vi "Actor Core.vi"(8 "error in":errorcluster, 11 "Analog Output Channel in":refnum<class "Analog Output Channel.lvclass">) -> (0 "error out":errorcluster, 3 "Actor out":refnum<class "Actor.lvclass">)   [LabVIEW 2015, in "Analog Output Channel.lvlib" / "Analog Output Channel.lvclass"]
doc: "(<B>Filename</B>: Actor Framework.lvlib:Actor.lvclass:Actor Core.vi)\n\nReceives messages to the actor, reacts to them, and initiates any error handling that may shut the actor down.\n\nDescendant classes may override this VI to append parallel tasks for the actor to complete while it handles messages. Overrides use the Call Parent Method node."
uses:
  Analog Output Channel.lvclass
  <vilib>/ActorFramework/Actor/Actor.lvclass
  <vilib>/ActorFramework/Actor/Actor.lvclass/Actor.ctl
  <vilib>/ActorFramework/Message Enqueuer/Message Enqueuer.lvclass/Message Enqueuer.ctl
  <userlib>/_Win8uiFramework/ViewableActor.lvclass/ViewableActor.ctl
  AOChData.lvclass
  <userlib>/_Win8uiFramework/Read Stop Event.vi
  <vilib>/ActorFramework/Message Enqueuer/Init from Existing Queue.vi
  <vilib>/ActorFramework/Message Enqueuer/Message Enqueuer.lvclass
  Channel/ChannelInfo.lvclass
  Channel/ChannelData.lvclass
  Channel/ChannelConfig.lvclass
  Output Channel/Output Channel/Output Channel.lvclass
  <userlib>/_Win8uiFramework/ViewableActor.lvclass
  <userlib>/_Win8uiFramework/Win8uiFramework.lvlib
  Analog Output Channel Messages/Write Sine Wave Msg/Write Sine Wave Msg.lvclass
panel:
  out "size(s)":i32
  in  "String":string
  out "Waveform Graph":dbl[](graph)
  in  "Write Sine Wave":bool
  in  "Sine Wave Parameters":T1={"phase"=0.0, "amplitude"=1.0, "frequency"=10.0, "offset"=0.0} {"offset" format="%#_13g"; "frequency" format="%0.2p"; "amplitude" format="%0.2p"; "phase" format="%.2p"}
  out "Sequence Parameters":cluster{"Buffer Size":dbl, "Sample Rate":dbl}
  out "Device Address":tag
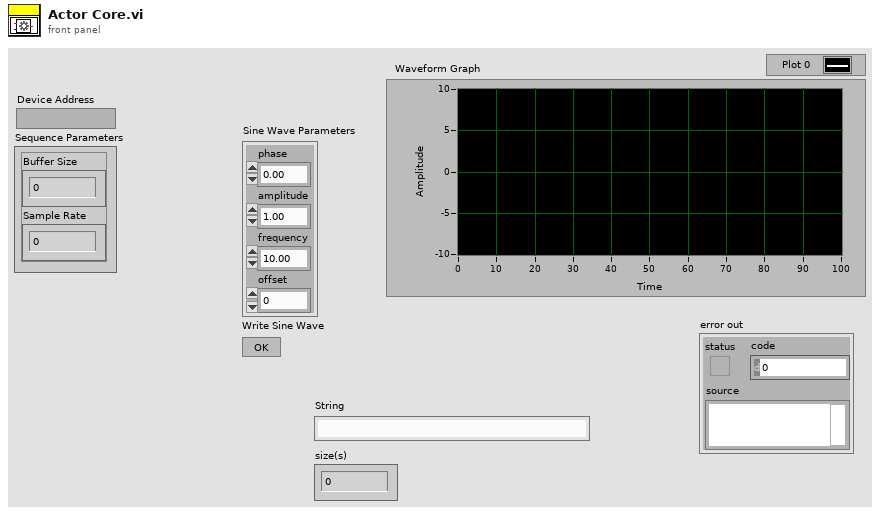
[diagram p1: front panel]
types:
  T1 = cluster{"phase":dbl, "amplitude":dbl, "frequency":dbl, "offset":dbl}
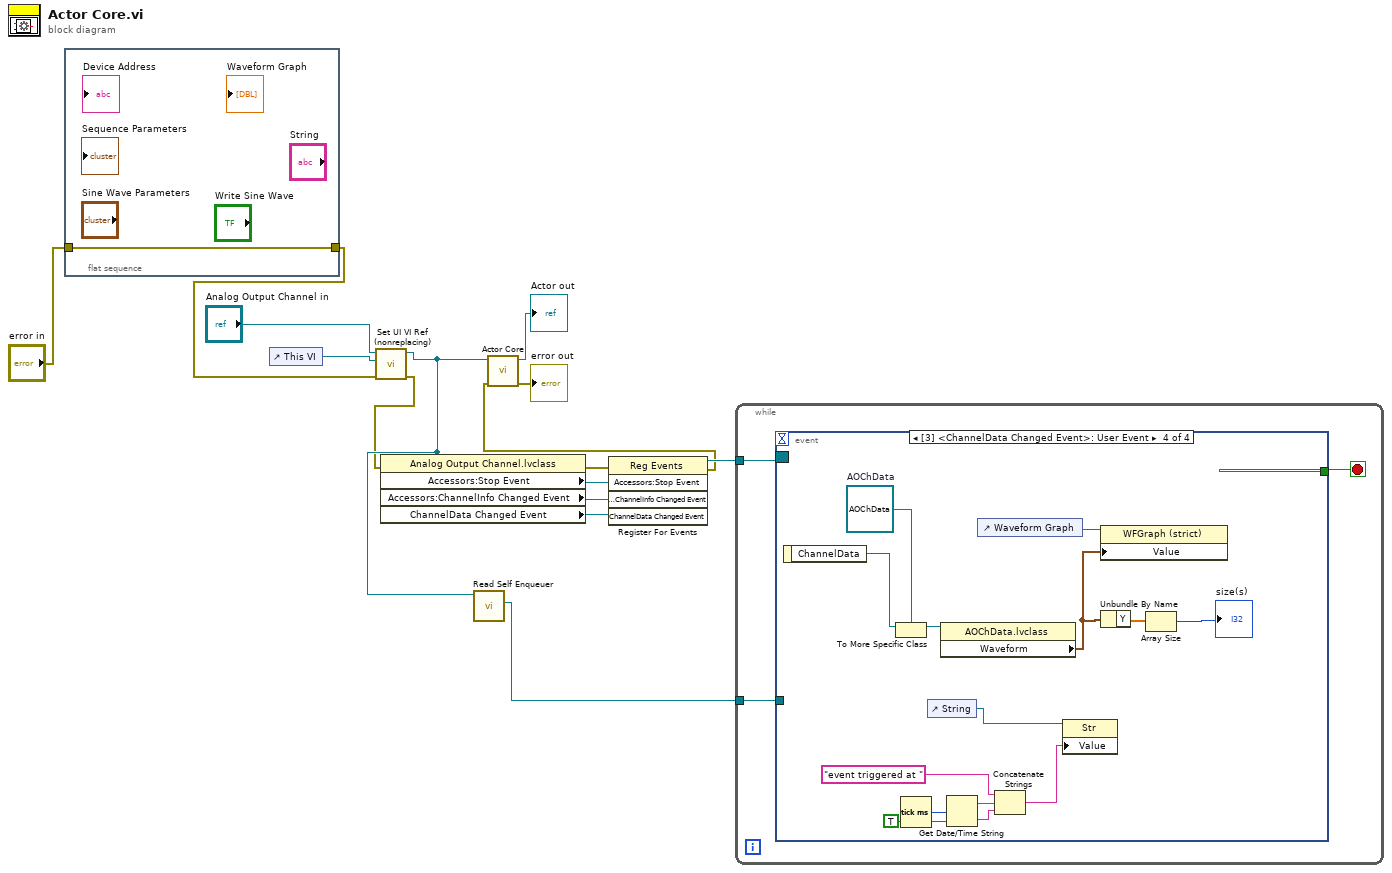
[diagram p0: block diagram]
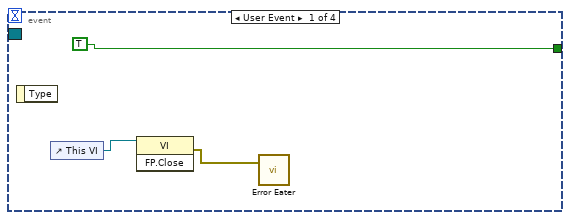
[diagram p2: hidden frame]
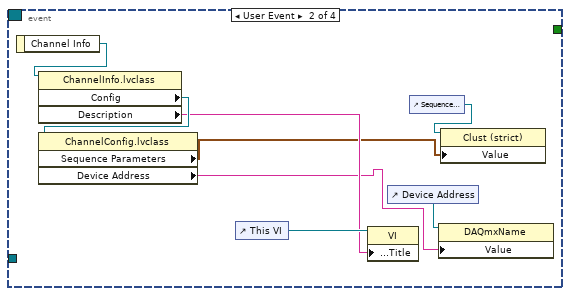
[diagram p3: hidden frame]
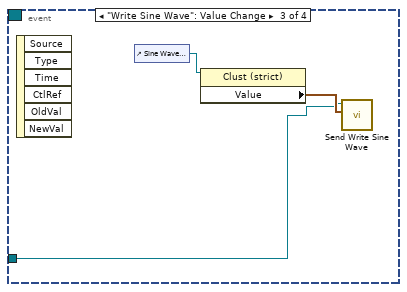
[diagram p4: hidden frame]
diagram:
  n1 = flat-sequence {
    tunnel: "error in" -> [w16]
    tunnel: [w16] -> w1
    frame #0 {
    }
  }
  n2 = control-ref of="This VI"() -> (w13:refnum<vi>)
  n3 = call <userlib>:"Set UI VI Ref (nonreplacing).vi"("error in (no error)"=w1, "UI VI Ref"=w13, "ViewableActor in"="Analog Output Channel in") -> ("error out"=w5:errorcluster, "ViewableActor out"=w8:refnum<class "Analog Output Channel.lvclass">)  [unwired: 6 in, 1 out]
  n4 = property class="Analog Output Channel.lvclass"(reference=w8, error in=w5) -> (error out=w4:errorcluster, "Accessors:Stop Event"=w11:refnum<user-event>, "Accessors:ChannelInfo Changed Event"=w10:refnum<user-event>, "ChannelData Changed Event"=w6:refnum<user-event>)  [unwired: 1 out]
  n5 = call <vilib>:"Read Self Enqueuer.vi"("Actor"=w8) -> ("Self Enqueuer"=w7:refnum<class "Message Enqueuer.lvclass">)  [unwired: 10 in]
  n6 = register-events(error in=w4, w11, w10, w6) -> (reference out=w9:refnum<event-registration>, error out=w3:errorcluster)  [unwired: 1 in]
  n7 = call-parent "Actor Core.vi"("error in"=w3, "Channel in"=w8) -> ("error out"=→"error out":errorcluster, "Actor out"=→"Actor out":refnum<class "Actor.lvclass">)  [unwired: 8 in]
  n8 = while {
    tunnel: w9 -> [w19]
    tunnel: w7 -> [w17]
    stop <- w18 stop-if-true
    n9 = event shown="[3] <ChannelData Changed Event>: User Event" {
      selector: w19 -> [_ _ _ _]
      dyn-events: _ -> [_ _ _ _]
      timeout: _ -> [_ _ _ _]
      tunnel: [TRUE _ _ _] -> w18
      tunnel: w17 -> [_ _ w32 _]
      event User Event {
        n10 = event-data() -> ()  [unwired: 1 in, 1 out]
        n11 = control-ref of="This VI"() -> (w21:refnum<vi>)
        n12 = invoke class="VI" method="FP.Close"(reference=w21) -> (error out=w20:errorcluster)  [unwired: 2 in, 2 out]
        n13 = call <userlib>:"Error Eater.vi"("error in (no error)"=w20) -> ()  [unwired: 2 in]
      }
      event User Event {
        n14 = event-data() -> ("Channel Info"=w27:refnum<class "ChannelInfo.lvclass">)  [unwired: 1 in]
        n15 = property class="ChannelInfo.lvclass"(reference=w27) -> ("Config"=w30:refnum<class "ChannelConfig.lvclass">, "Description"=w28:string)  [unwired: 1 in, 2 out]
        n16 = property class="ChannelConfig.lvclass"(reference=w30) -> ("Sequence Parameters"=w25:cluster{"Buffer Size":dbl, "Sample Rate":dbl}, "Device Address"=w23:tag)  [unwired: 1 in, 2 out]
        n17 = control-ref of="This VI"() -> (w29:refnum<vi>)
        n18 = property class="VI"(reference=w29, "Front Panel.Title"=w28) -> ()  [unwired: 1 in, 2 out]
        n19 = control-ref of="Device Address"() -> (w24:refnum<vi>)
        n20 = control-ref of="Sequence Parameters"() -> (w26:refnum<vi>)
        n21 = property class="DAQmxName"(reference=w24, "Value"=w23) -> ()  [unwired: 1 in, 2 out]
        n22 = property class="Clust (strict)"(reference=w26, "Value"=w25) -> ()  [unwired: 1 in, 2 out]
      }
      event "Write Sine Wave": Value Change {
        n23 = event-data() -> ()  [unwired: 1 in, 6 out]
        n24 = control-ref of="Sine Wave Parameters"() -> (w31:refnum<vi>)
        n25 = property class="Clust (strict)"(reference=w31) -> ("Value"=w33:T1)  [unwired: 1 in, 2 out]
        n26 = call "Send Write Sine Wave.vi"("Sin Wave Parameters"=w33, "Message Enqueuer in"=w32) -> ()  [unwired: 8 in, 2 out]
      }
      event User Event {
        w46 = refnum<class "AOChData.lvclass"> refnum  # AOChData
        n27 = event-data() -> ("ChannelData"=w45:refnum<class "ChannelData.lvclass">)  [unwired: 1 in]
        n28 = To More Specific Class(target class=w46, reference=w45) -> (specific class reference=w44:refnum<class "AOChData.lvclass">)  [unwired: 1 in, 1 out]
        n29 = Tick Count (ms)() -> (millisecond timer value=w42:u32)
        n30 = control-ref of="String"() -> (w43:refnum<vi>)
        n31 = property class="AOChData.lvclass"(reference=w44) -> ("Waveform"=w36:waveform(dbl))  [unwired: 1 in, 2 out]
        n32 = Get Date/Time String(seconds (now)=w42, want seconds? (F)=TRUE) -> (date string=w41:string, time string=w40:string)  [unwired: 1 in]
        n33 = control-ref of="Waveform Graph"() -> (w47:refnum<vi>)
        n34 = Concatenate Strings("event triggered at " ("Description"), w41, w40) -> (w37:string)
        n35 = property class="Str"(reference=w43, "Value"=w37) -> ()  [unwired: 1 in, 2 out]
        n36 = property class="WFGraph (strict)"(reference=w47, "Value"=w36) -> ()  [unwired: 1 in, 2 out]
        n37 = Unbundle By Name(w36) -> ("Y"=w35:dbl[])
        n38 = Array Size(array=w35) -> (size(s)=→"size(s)":i32)
      }
    }
  }
